vi "AD7609 Check overrun.vi"() -> (1 "Overruns":u32, 2 "Overrun error out":errorcluster)   [LabVIEW 2015]
uses:
  <vilib>/Instr/_visa.llb/VISA Open Access Mode.ctl
  AD7609 global.vi
panel:
  out "Overrun string output":string
  # "PN 25/11/2014, 17/08/2015"
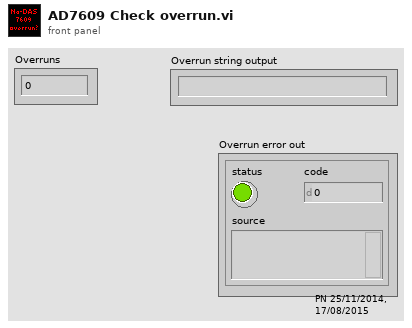
[diagram p1: front panel]
types:
  T1 = typedef "VISA Open Access Mode.ctl" = u32
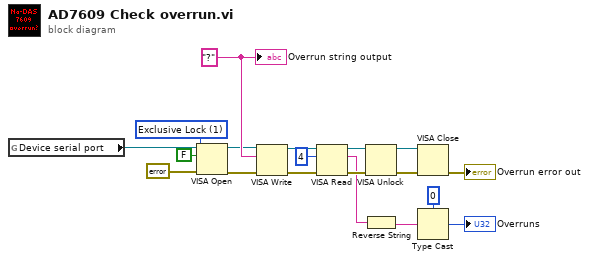
[diagram p0: block diagram]
diagram:
  w19 = T1 1 items=["VISA Defaults"=0, "Exclusive Lock"=1, "Load Configured Settings"=4] ("Access Mode")
  w12 = "?"
  n1 = global read "AD7609 global.vi" "Device serial port"() -> (w13:refnum<visa-resource-name>)
  n2 = VISA Open(duplicate session (F)=FALSE, access mode=w19, error in (no error)=errorcluster {"status"=FALSE, "code"=0, "source"=""}, VISA resource name=w13) -> (VISA resource name=w2:refnum<visa-resource-name>, error out=w1:errorcluster)  [unwired: 1 in]
  n3 = VISA Write(VISA resource name=w2, write buffer=w12, error in (no error)=w1) -> (VISA resource name out=w8:refnum<visa-resource-name>, error out=w11:errorcluster)  [unwired: 1 out]
  n4 = VISA Read(VISA resource name=w8, byte count=u32 4, error in (no error)=w11) -> (VISA resource name out=w7:refnum<visa-resource-name>, read buffer=w5:string, error out=w10:errorcluster)  [unwired: 1 out]
  n5 = VISA Unlock(8:w10, 11:w7) -> (0:w16:errorcluster, 3:w17:refnum<visa-resource-name>)
  n6 = Reverse String(1:w5) -> (0:w3:string)
  n7 = VISA Close(VISA resource name=w17, error in (no error)=w16) -> (error out=→"Overrun error out":errorcluster)
  n8 = Type Cast(type=u32 0, x=w3) -> (*(type *) &x=→"Overruns":u32)
  "Overrun string output" <- w12
